vi "数字量输出配置.vi"() -> ()   [LabVIEW 2010] (continued)
            }
            frame 65 {
              w158 = TRUE
              w159 = FALSE ("单选_第41路")
              n5551 = local write "单选_第1路"(w158) -> ()
              n5552 = local write "单选_第2路"(w158) -> ()
              n5553 = local write "单选_第3路"(w158) -> ()
              n5554 = local write "单选_第4路"(w158) -> ()
              n5555 = local write "单选_第5路"(w158) -> ()
              n5556 = local write "单选_第6路"(w158) -> ()
              n5557 = local write "单选_第7路"(w158) -> ()
              n5558 = local write "单选_第8路"(w158) -> ()
              n5559 = local write "单选_第9路"(w158) -> ()
              n5560 = local write "单选_第10路"(w158) -> ()
              n5561 = local write "单选_第11路"(w158) -> ()
              n5562 = local write "单选_第12路"(w158) -> ()
              n5563 = local write "单选_第13路"(w158) -> ()
              n5564 = local write "单选_第14路"(w158) -> ()
              n5565 = local write "单选_第15路"(w158) -> ()
              n5566 = local write "单选_第16路"(w158) -> ()
              n5567 = local write "单选_第17路"(w158) -> ()
              n5568 = local write "单选_第18路"(w158) -> ()
              n5569 = local write "单选_第19路"(w158) -> ()
              n5570 = local write "单选_第20路"(w158) -> ()
              n5571 = local write "单选_第21路"(w158) -> ()
              n5572 = local write "单选_第22路"(w158) -> ()
              n5573 = local write "单选_第23路"(w158) -> ()
              n5574 = local write "单选_第24路"(w158) -> ()
              n5575 = local write "单选_第25路"(w158) -> ()
              n5576 = local write "单选_第26路"(w158) -> ()
              n5577 = local write "单选_第27路"(w158) -> ()
              n5578 = local write "单选_第28路"(w158) -> ()
              n5579 = local write "单选_第29路"(w158) -> ()
              n5580 = local write "单选_第30路"(w158) -> ()
              n5581 = local write "单选_第31路"(w158) -> ()
              n5582 = local write "单选_第32路"(w158) -> ()
              n5583 = local write "单选_第33路"(w158) -> ()
              n5584 = local write "单选_第34路"(w158) -> ()
              n5585 = local write "单选_第35路"(w158) -> ()
              n5586 = local write "单选_第36路"(w158) -> ()
              n5587 = local write "单选_第37路"(w158) -> ()
              n5588 = local write "单选_第38路"(w158) -> ()
              n5589 = local write "单选_第39路"(w158) -> ()
              n5590 = local write "单选_第40路"(w158) -> ()
              n5591 = local write "单选_第41路"(w158) -> ()
              n5592 = local write "单选_第42路"(w158) -> ()
              n5593 = local write "单选_第43路"(w158) -> ()
              n5594 = local write "单选_第44路"(w158) -> ()
              n5595 = local write "单选_第45路"(w158) -> ()
              n5596 = local write "单选_第46路"(w158) -> ()
              n5597 = local write "单选_第47路"(w158) -> ()
              n5598 = local write "单选_第48路"(w158) -> ()
              n5599 = local write "单选_第49路"(w158) -> ()
              n5600 = local write "单选_第50路"(w158) -> ()
              n5601 = local write "单选_第51路"(w158) -> ()
              n5602 = local write "单选_第52路"(w158) -> ()
              n5603 = local write "单选_第53路"(w158) -> ()
              n5604 = local write "单选_第54路"(w158) -> ()
              n5605 = local write "单选_第55路"(w158) -> ()
              n5606 = local write "单选_第56路"(w158) -> ()
              n5607 = local write "单选_第57路"(w158) -> ()
              n5608 = local write "单选_第58路"(w158) -> ()
              n5609 = local write "单选_第59路"(w158) -> ()
              n5610 = local write "单选_第60路"(w158) -> ()
              n5611 = local write "单选_第71路"(w159) -> ()
              n5612 = local write "单选_第79路"(w159) -> ()
              n5613 = local write "单选_第65路"(w158) -> ()
              n5614 = local write "单选_第66路"(w158) -> ()
              n5615 = local write "单选_第67路"(w158) -> ()
              n5616 = local write "单选_第68路"(w158) -> ()
              n5617 = local write "单选_第69路"(w158) -> ()
              n5618 = local write "单选_第70路"(w159) -> ()
              n5619 = local write "单选_第72路"(w159) -> ()
              n5620 = local write "单选_第73路"(w159) -> ()
              n5621 = local write "单选_第74路"(w159) -> ()
              n5622 = local write "单选_第75路"(w159) -> ()
              n5623 = local write "单选_第76路"(w159) -> ()
              n5624 = local write "单选_第77路"(w159) -> ()
              n5625 = local write "单选_第78路"(w159) -> ()
              n5626 = local write "单选_第80路"(w159) -> ()
            }
            frame 66 {
              w160 = TRUE
              w161 = FALSE ("单选_第41路")
              n5627 = local write "单选_第1路"(w160) -> ()
              n5628 = local write "单选_第2路"(w160) -> ()
              n5629 = local write "单选_第3路"(w160) -> ()
              n5630 = local write "单选_第4路"(w160) -> ()
              n5631 = local write "单选_第5路"(w160) -> ()
              n5632 = local write "单选_第6路"(w160) -> ()
              n5633 = local write "单选_第7路"(w160) -> ()
              n5634 = local write "单选_第8路"(w160) -> ()
              n5635 = local write "单选_第9路"(w160) -> ()
              n5636 = local write "单选_第10路"(w160) -> ()
              n5637 = local write "单选_第11路"(w160) -> ()
              n5638 = local write "单选_第12路"(w160) -> ()
              n5639 = local write "单选_第13路"(w160) -> ()
              n5640 = local write "单选_第14路"(w160) -> ()
              n5641 = local write "单选_第15路"(w160) -> ()
              n5642 = local write "单选_第16路"(w160) -> ()
              n5643 = local write "单选_第17路"(w160) -> ()
              n5644 = local write "单选_第18路"(w160) -> ()
              n5645 = local write "单选_第19路"(w160) -> ()
              n5646 = local write "单选_第20路"(w160) -> ()
              n5647 = local write "单选_第21路"(w160) -> ()
              n5648 = local write "单选_第22路"(w160) -> ()
              n5649 = local write "单选_第23路"(w160) -> ()
              n5650 = local write "单选_第24路"(w160) -> ()
              n5651 = local write "单选_第25路"(w160) -> ()
              n5652 = local write "单选_第26路"(w160) -> ()
              n5653 = local write "单选_第27路"(w160) -> ()
              n5654 = local write "单选_第28路"(w160) -> ()
              n5655 = local write "单选_第29路"(w160) -> ()
              n5656 = local write "单选_第30路"(w160) -> ()
              n5657 = local write "单选_第31路"(w160) -> ()
              n5658 = local write "单选_第32路"(w160) -> ()
              n5659 = local write "单选_第33路"(w160) -> ()
              n5660 = local write "单选_第34路"(w160) -> ()
              n5661 = local write "单选_第35路"(w160) -> ()
              n5662 = local write "单选_第36路"(w160) -> ()
              n5663 = local write "单选_第37路"(w160) -> ()
              n5664 = local write "单选_第38路"(w160) -> ()
              n5665 = local write "单选_第39路"(w160) -> ()
              n5666 = local write "单选_第40路"(w160) -> ()
              n5667 = local write "单选_第41路"(w160) -> ()
              n5668 = local write "单选_第42路"(w160) -> ()
              n5669 = local write "单选_第43路"(w160) -> ()
              n5670 = local write "单选_第44路"(w160) -> ()
              n5671 = local write "单选_第45路"(w160) -> ()
              n5672 = local write "单选_第46路"(w160) -> ()
              n5673 = local write "单选_第47路"(w160) -> ()
              n5674 = local write "单选_第48路"(w160) -> ()
              n5675 = local write "单选_第49路"(w160) -> ()
              n5676 = local write "单选_第50路"(w160) -> ()
              n5677 = local write "单选_第51路"(w160) -> ()
              n5678 = local write "单选_第52路"(w160) -> ()
              n5679 = local write "单选_第53路"(w160) -> ()
              n5680 = local write "单选_第54路"(w160) -> ()
              n5681 = local write "单选_第55路"(w160) -> ()
              n5682 = local write "单选_第56路"(w160) -> ()
              n5683 = local write "单选_第57路"(w160) -> ()
              n5684 = local write "单选_第58路"(w160) -> ()
              n5685 = local write "单选_第59路"(w160) -> ()
              n5686 = local write "单选_第60路"(w160) -> ()
              n5687 = local write "单选_第71路"(w161) -> ()
              n5688 = local write "单选_第79路"(w161) -> ()
              n5689 = local write "单选_第65路"(w160) -> ()
              n5690 = local write "单选_第66路"(w160) -> ()
              n5691 = local write "单选_第67路"(w160) -> ()
              n5692 = local write "单选_第68路"(w160) -> ()
              n5693 = local write "单选_第69路"(w160) -> ()
              n5694 = local write "单选_第70路"(w160) -> ()
              n5695 = local write "单选_第72路"(w161) -> ()
              n5696 = local write "单选_第73路"(w161) -> ()
              n5697 = local write "单选_第74路"(w161) -> ()
              n5698 = local write "单选_第75路"(w161) -> ()
              n5699 = local write "单选_第76路"(w161) -> ()
              n5700 = local write "单选_第77路"(w161) -> ()
              n5701 = local write "单选_第78路"(w161) -> ()
              n5702 = local write "单选_第80路"(w161) -> ()
            }
            frame 67 {
              w162 = TRUE
              w163 = FALSE ("单选_第41路")
              n5703 = local write "单选_第1路"(w162) -> ()
              n5704 = local write "单选_第2路"(w162) -> ()
              n5705 = local write "单选_第3路"(w162) -> ()
              n5706 = local write "单选_第4路"(w162) -> ()
              n5707 = local write "单选_第5路"(w162) -> ()
              n5708 = local write "单选_第6路"(w162) -> ()
              n5709 = local write "单选_第7路"(w162) -> ()
              n5710 = local write "单选_第8路"(w162) -> ()
              n5711 = local write "单选_第9路"(w162) -> ()
              n5712 = local write "单选_第10路"(w162) -> ()
              n5713 = local write "单选_第11路"(w162) -> ()
              n5714 = local write "单选_第12路"(w162) -> ()
              n5715 = local write "单选_第13路"(w162) -> ()
              n5716 = local write "单选_第14路"(w162) -> ()
              n5717 = local write "单选_第15路"(w162) -> ()
              n5718 = local write "单选_第16路"(w162) -> ()
              n5719 = local write "单选_第17路"(w162) -> ()
              n5720 = local write "单选_第18路"(w162) -> ()
              n5721 = local write "单选_第19路"(w162) -> ()
              n5722 = local write "单选_第20路"(w162) -> ()
              n5723 = local write "单选_第21路"(w162) -> ()
              n5724 = local write "单选_第22路"(w162) -> ()
              n5725 = local write "单选_第23路"(w162) -> ()
              n5726 = local write "单选_第24路"(w162) -> ()
              n5727 = local write "单选_第25路"(w162) -> ()
              n5728 = local write "单选_第26路"(w162) -> ()
              n5729 = local write "单选_第27路"(w162) -> ()
              n5730 = local write "单选_第28路"(w162) -> ()
              n5731 = local write "单选_第29路"(w162) -> ()
              n5732 = local write "单选_第30路"(w162) -> ()
              n5733 = local write "单选_第31路"(w162) -> ()
              n5734 = local write "单选_第32路"(w162) -> ()
              n5735 = local write "单选_第33路"(w162) -> ()
              n5736 = local write "单选_第34路"(w162) -> ()
              n5737 = local write "单选_第35路"(w162) -> ()
              n5738 = local write "单选_第36路"(w162) -> ()
              n5739 = local write "单选_第37路"(w162) -> ()
              n5740 = local write "单选_第38路"(w162) -> ()
              n5741 = local write "单选_第39路"(w162) -> ()
              n5742 = local write "单选_第40路"(w162) -> ()
              n5743 = local write "单选_第41路"(w162) -> ()
              n5744 = local write "单选_第42路"(w162) -> ()
              n5745 = local write "单选_第43路"(w162) -> ()
              n5746 = local write "单选_第44路"(w162) -> ()
              n5747 = local write "单选_第45路"(w162) -> ()
              n5748 = local write "单选_第46路"(w162) -> ()
              n5749 = local write "单选_第47路"(w162) -> ()
              n5750 = local write "单选_第48路"(w162) -> ()
              n5751 = local write "单选_第49路"(w162) -> ()
              n5752 = local write "单选_第50路"(w162) -> ()
              n5753 = local write "单选_第51路"(w162) -> ()
              n5754 = local write "单选_第52路"(w162) -> ()
              n5755 = local write "单选_第53路"(w162) -> ()
              n5756 = local write "单选_第54路"(w162) -> ()
              n5757 = local write "单选_第55路"(w162) -> ()
              n5758 = local write "单选_第56路"(w162) -> ()
              n5759 = local write "单选_第57路"(w162) -> ()
              n5760 = local write "单选_第58路"(w162) -> ()
              n5761 = local write "单选_第59路"(w162) -> ()
              n5762 = local write "单选_第60路"(w162) -> ()
              n5763 = local write "单选_第71路"(w162) -> ()
              n5764 = local write "单选_第79路"(w163) -> ()
              n5765 = local write "单选_第65路"(w162) -> ()
              n5766 = local write "单选_第66路"(w162) -> ()
              n5767 = local write "单选_第67路"(w162) -> ()
              n5768 = local write "单选_第68路"(w162) -> ()
              n5769 = local write "单选_第69路"(w162) -> ()
              n5770 = local write "单选_第70路"(w162) -> ()
              n5771 = local write "单选_第72路"(w163) -> ()
              n5772 = local write "单选_第73路"(w163) -> ()
              n5773 = local write "单选_第74路"(w163) -> ()
              n5774 = local write "单选_第75路"(w163) -> ()
              n5775 = local write "单选_第76路"(w163) -> ()
              n5776 = local write "单选_第77路"(w163) -> ()
              n5777 = local write "单选_第78路"(w163) -> ()
              n5778 = local write "单选_第80路"(w163) -> ()
            }
            frame 68 {
              w164 = TRUE
              w165 = FALSE ("单选_第41路")
              n5779 = local write "单选_第1路"(w164) -> ()
              n5780 = local write "单选_第2路"(w164) -> ()
              n5781 = local write "单选_第3路"(w164) -> ()
              n5782 = local write "单选_第4路"(w164) -> ()
              n5783 = local write "单选_第5路"(w164) -> ()
              n5784 = local write "单选_第6路"(w164) -> ()
              n5785 = local write "单选_第7路"(w164) -> ()
              n5786 = local write "单选_第8路"(w164) -> ()
              n5787 = local write "单选_第9路"(w164) -> ()
              n5788 = local write "单选_第10路"(w164) -> ()
              n5789 = local write "单选_第11路"(w164) -> ()
              n5790 = local write "单选_第12路"(w164) -> ()
              n5791 = local write "单选_第13路"(w164) -> ()
              n5792 = local write "单选_第14路"(w164) -> ()
              n5793 = local write "单选_第15路"(w164) -> ()
              n5794 = local write "单选_第16路"(w164) -> ()
              n5795 = local write "单选_第17路"(w164) -> ()
              n5796 = local write "单选_第18路"(w164) -> ()
              n5797 = local write "单选_第19路"(w164) -> ()
              n5798 = local write "单选_第20路"(w164) -> ()
              n5799 = local write "单选_第21路"(w164) -> ()
              n5800 = local write "单选_第22路"(w164) -> ()
              n5801 = local write "单选_第23路"(w164) -> ()
              n5802 = local write "单选_第24路"(w164) -> ()
              n5803 = local write "单选_第25路"(w164) -> ()
              n5804 = local write "单选_第26路"(w164) -> ()
              n5805 = local write "单选_第27路"(w164) -> ()
              n5806 = local write "单选_第28路"(w164) -> ()
              n5807 = local write "单选_第29路"(w164) -> ()
              n5808 = local write "单选_第30路"(w164) -> ()
              n5809 = local write "单选_第31路"(w164) -> ()
              n5810 = local write "单选_第32路"(w164) -> ()
              n5811 = local write "单选_第33路"(w164) -> ()
              n5812 = local write "单选_第34路"(w164) -> ()
              n5813 = local write "单选_第35路"(w164) -> ()
              n5814 = local write "单选_第36路"(w164) -> ()
              n5815 = local write "单选_第37路"(w164) -> ()
              n5816 = local write "单选_第38路"(w164) -> ()
              n5817 = local write "单选_第39路"(w164) -> ()
              n5818 = local write "单选_第40路"(w164) -> ()
              n5819 = local write "单选_第41路"(w164) -> ()
              n5820 = local write "单选_第42路"(w164) -> ()
              n5821 = local write "单选_第43路"(w164) -> ()
              n5822 = local write "单选_第44路"(w164) -> ()
              n5823 = local write "单选_第45路"(w164) -> ()
              n5824 = local write "单选_第46路"(w164) -> ()
              n5825 = local write "单选_第47路"(w164) -> ()
              n5826 = local write "单选_第48路"(w164) -> ()
              n5827 = local write "单选_第49路"(w164) -> ()
              n5828 = local write "单选_第50路"(w164) -> ()
              n5829 = local write "单选_第51路"(w164) -> ()
              n5830 = local write "单选_第52路"(w164) -> ()
              n5831 = local write "单选_第53路"(w164) -> ()
              n5832 = local write "单选_第54路"(w164) -> ()
              n5833 = local write "单选_第55路"(w164) -> ()
              n5834 = local write "单选_第56路"(w164) -> ()
              n5835 = local write "单选_第57路"(w164) -> ()
              n5836 = local write "单选_第58路"(w164) -> ()
              n5837 = local write "单选_第59路"(w164) -> ()
              n5838 = local write "单选_第60路"(w164) -> ()
              n5839 = local write "单选_第71路"(w164) -> ()
              n5840 = local write "单选_第79路"(w165) -> ()
              n5841 = local write "单选_第65路"(w164) -> ()
              n5842 = local write "单选_第66路"(w164) -> ()
              n5843 = local write "单选_第67路"(w164) -> ()
              n5844 = local write "单选_第68路"(w164) -> ()
              n5845 = local write "单选_第69路"(w164) -> ()
              n5846 = local write "单选_第70路"(w164) -> ()
              n5847 = local write "单选_第72路"(w164) -> ()
              n5848 = local write "单选_第73路"(w165) -> ()
              n5849 = local write "单选_第74路"(w165) -> ()
              n5850 = local write "单选_第75路"(w165) -> ()
              n5851 = local write "单选_第76路"(w165) -> ()
              n5852 = local write "单选_第77路"(w165) -> ()
              n5853 = local write "单选_第78路"(w165) -> ()
              n5854 = local write "单选_第80路"(w165) -> ()
            }
            frame 69 {
              w166 = TRUE
              w167 = FALSE ("单选_第41路")
              n5855 = local write "单选_第1路"(w166) -> ()
              n5856 = local write "单选_第2路"(w166) -> ()
              n5857 = local write "单选_第3路"(w166) -> ()
              n5858 = local write "单选_第4路"(w166) -> ()
              n5859 = local write "单选_第5路"(w166) -> ()
              n5860 = local write "单选_第6路"(w166) -> ()
              n5861 = local write "单选_第7路"(w166) -> ()
              n5862 = local write "单选_第8路"(w166) -> ()
              n5863 = local write "单选_第9路"(w166) -> ()
              n5864 = local write "单选_第10路"(w166) -> ()
              n5865 = local write "单选_第11路"(w166) -> ()
              n5866 = local write "单选_第12路"(w166) -> ()
              n5867 = local write "单选_第13路"(w166) -> ()
              n5868 = local write "单选_第14路"(w166) -> ()
              n5869 = local write "单选_第15路"(w166) -> ()
              n5870 = local write "单选_第16路"(w166) -> ()
              n5871 = local write "单选_第17路"(w166) -> ()
              n5872 = local write "单选_第18路"(w166) -> ()
              n5873 = local write "单选_第19路"(w166) -> ()
              n5874 = local write "单选_第20路"(w166) -> ()
              n5875 = local write "单选_第21路"(w166) -> ()
              n5876 = local write "单选_第22路"(w166) -> ()
              n5877 = local write "单选_第23路"(w166) -> ()
              n5878 = local write "单选_第24路"(w166) -> ()
              n5879 = local write "单选_第25路"(w166) -> ()
              n5880 = local write "单选_第26路"(w166) -> ()
              n5881 = local write "单选_第27路"(w166) -> ()
              n5882 = local write "单选_第28路"(w166) -> ()
              n5883 = local write "单选_第29路"(w166) -> ()
              n5884 = local write "单选_第30路"(w166) -> ()
              n5885 = local write "单选_第31路"(w166) -> ()
              n5886 = local write "单选_第32路"(w166) -> ()
              n5887 = local write "单选_第33路"(w166) -> ()
              n5888 = local write "单选_第34路"(w166) -> ()
              n5889 = local write "单选_第35路"(w166) -> ()
              n5890 = local write "单选_第36路"(w166) -> ()
              n5891 = local write "单选_第37路"(w166) -> ()
              n5892 = local write "单选_第38路"(w166) -> ()
              n5893 = local write "单选_第39路"(w166) -> ()
              n5894 = local write "单选_第40路"(w166) -> ()
              n5895 = local write "单选_第41路"(w166) -> ()
              n5896 = local write "单选_第42路"(w166) -> ()
              n5897 = local write "单选_第43路"(w166) -> ()
              n5898 = local write "单选_第44路"(w166) -> ()
              n5899 = local write "单选_第45路"(w166) -> ()
              n5900 = local write "单选_第46路"(w166) -> ()
              n5901 = local write "单选_第47路"(w166) -> ()
              n5902 = local write "单选_第48路"(w166) -> ()
              n5903 = local write "单选_第49路"(w166) -> ()
              n5904 = local write "单选_第50路"(w166) -> ()
              n5905 = local write "单选_第51路"(w166) -> ()
              n5906 = local write "单选_第52路"(w166) -> ()
              n5907 = local write "单选_第53路"(w166) -> ()
              n5908 = local write "单选_第54路"(w166) -> ()
              n5909 = local write "单选_第55路"(w166) -> ()
              n5910 = local write "单选_第56路"(w166) -> ()
              n5911 = local write "单选_第57路"(w166) -> ()
              n5912 = local write "单选_第58路"(w166) -> ()
              n5913 = local write "单选_第59路"(w166) -> ()
              n5914 = local write "单选_第60路"(w166) -> ()
              n5915 = local write "单选_第71路"(w166) -> ()
              n5916 = local write "单选_第79路"(w167) -> ()
              n5917 = local write "单选_第65路"(w166) -> ()
              n5918 = local write "单选_第66路"(w166) -> ()
              n5919 = local write "单选_第67路"(w166) -> ()
              n5920 = local write "单选_第68路"(w166) -> ()
              n5921 = local write "单选_第69路"(w166) -> ()
              n5922 = local write "单选_第70路"(w166) -> ()
              n5923 = local write "单选_第72路"(w166) -> ()
              n5924 = local write "单选_第73路"(w166) -> ()
              n5925 = local write "单选_第74路"(w167) -> ()
              n5926 = local write "单选_第75路"(w167) -> ()
              n5927 = local write "单选_第76路"(w167) -> ()
              n5928 = local write "单选_第77路"(w167) -> ()
              n5929 = local write "单选_第78路"(w167) -> ()
              n5930 = local write "单选_第80路"(w167) -> ()
            }
            frame 70 {
              w168 = TRUE
              w169 = FALSE ("单选_第41路")
              n5931 = local write "单选_第1路"(w168) -> ()
              n5932 = local write "单选_第2路"(w168) -> ()
              n5933 = local write "单选_第3路"(w168) -> ()
              n5934 = local write "单选_第4路"(w168) -> ()
              n5935 = local write "单选_第5路"(w168) -> ()
              n5936 = local write "单选_第6路"(w168) -> ()
              n5937 = local write "单选_第7路"(w168) -> ()
              n5938 = local write "单选_第8路"(w168) -> ()
              n5939 = local write "单选_第9路"(w168) -> ()
              n5940 = local write "单选_第10路"(w168) -> ()
              n5941 = local write "单选_第11路"(w168) -> ()
              n5942 = local write "单选_第12路"(w168) -> ()
              n5943 = local write "单选_第13路"(w168) -> ()
              n5944 = local write "单选_第14路"(w168) -> ()
              n5945 = local write "单选_第15路"(w168) -> ()
              n5946 = local write "单选_第16路"(w168) -> ()
              n5947 = local write "单选_第17路"(w168) -> ()
              n5948 = local write "单选_第18路"(w168) -> ()
              n5949 = local write "单选_第19路"(w168) -> ()
              n5950 = local write "单选_第20路"(w168) -> ()
              n5951 = local write "单选_第21路"(w168) -> ()
              n5952 = local write "单选_第22路"(w168) -> ()
              n5953 = local write "单选_第23路"(w168) -> ()
              n5954 = local write "单选_第24路"(w168) -> ()
              n5955 = local write "单选_第25路"(w168) -> ()
              n5956 = local write "单选_第26路"(w168) -> ()
              n5957 = local write "单选_第27路"(w168) -> ()
              n5958 = local write "单选_第28路"(w168) -> ()
              n5959 = local write "单选_第29路"(w168) -> ()
              n5960 = local write "单选_第30路"(w168) -> ()
              n5961 = local write "单选_第31路"(w168) -> ()
              n5962 = local write "单选_第32路"(w168) -> ()
              n5963 = local write "单选_第33路"(w168) -> ()
              n5964 = local write "单选_第34路"(w168) -> ()
              n5965 = local write "单选_第35路"(w168) -> ()
              n5966 = local write "单选_第36路"(w168) -> ()
              n5967 = local write "单选_第37路"(w168) -> ()
              n5968 = local write "单选_第38路"(w168) -> ()
              n5969 = local write "单选_第39路"(w168) -> ()
              n5970 = local write "单选_第40路"(w168) -> ()
              n5971 = local write "单选_第41路"(w168) -> ()
              n5972 = local write "单选_第42路"(w168) -> ()
              n5973 = local write "单选_第43路"(w168) -> ()
              n5974 = local write "单选_第44路"(w168) -> ()
              n5975 = local write "单选_第45路"(w168) -> ()
              n5976 = local write "单选_第46路"(w168) -> ()
              n5977 = local write "单选_第47路"(w168) -> ()
              n5978 = local write "单选_第48路"(w168) -> ()
              n5979 = local write "单选_第49路"(w168) -> ()
              n5980 = local write "单选_第50路"(w168) -> ()
              n5981 = local write "单选_第51路"(w168) -> ()
              n5982 = local write "单选_第52路"(w168) -> ()
              n5983 = local write "单选_第53路"(w168) -> ()
              n5984 = local write "单选_第54路"(w168) -> ()
              n5985 = local write "单选_第55路"(w168) -> ()
              n5986 = local write "单选_第56路"(w168) -> ()
              n5987 = local write "单选_第57路"(w168) -> ()
              n5988 = local write "单选_第58路"(w168) -> ()
              n5989 = local write "单选_第59路"(w168) -> ()
              n5990 = local write "单选_第60路"(w168) -> ()
              n5991 = local write "单选_第71路"(w168) -> ()
              n5992 = local write "单选_第79路"(w169) -> ()
              n5993 = local write "单选_第65路"(w168) -> ()
              n5994 = local write "单选_第66路"(w168) -> ()
              n5995 = local write "单选_第67路"(w168) -> ()
              n5996 = local write "单选_第68路"(w168) -> ()
              n5997 = local write "单选_第69路"(w168) -> ()
              n5998 = local write "单选_第70路"(w168) -> ()
              n5999 = local write "单选_第72路"(w168) -> ()
              n6000 = local write "单选_第73路"(w168) -> ()
              n6001 = local write "单选_第74路"(w168) -> ()
              n6002 = local write "单选_第75路"(w169) -> ()
              n6003 = local write "单选_第76路"(w169) -> ()
              n6004 = local write "单选_第77路"(w169) -> ()
              n6005 = local write "单选_第78路"(w169) -> ()
              n6006 = local write "单选_第80路"(w169) -> ()
            }
            frame 71 {
              w170 = TRUE
              w171 = FALSE ("单选_第41路")
              n6007 = local write "单选_第1路"(w170) -> ()
              n6008 = local write "单选_第2路"(w170) -> ()
              n6009 = local write "单选_第3路"(w170) -> ()
              n6010 = local write "单选_第4路"(w170) -> ()
              n6011 = local write "单选_第5路"(w170) -> ()
              n6012 = local write "单选_第6路"(w170) -> ()
              n6013 = local write "单选_第7路"(w170) -> ()
              n6014 = local write "单选_第8路"(w170) -> ()
              n6015 = local write "单选_第9路"(w170) -> ()
              n6016 = local write "单选_第10路"(w170) -> ()
              n6017 = local write "单选_第11路"(w170) -> ()
              n6018 = local write "单选_第12路"(w170) -> ()
              n6019 = local write "单选_第13路"(w170) -> ()
              n6020 = local write "单选_第14路"(w170) -> ()
              n6021 = local write "单选_第15路"(w170) -> ()
              n6022 = local write "单选_第16路"(w170) -> ()
              n6023 = local write "单选_第17路"(w170) -> ()
              n6024 = local write "单选_第18路"(w170) -> ()
              n6025 = local write "单选_第19路"(w170) -> ()
              n6026 = local write "单选_第20路"(w170) -> ()
              n6027 = local write "单选_第21路"(w170) -> ()
              n6028 = local write "单选_第22路"(w170) -> ()
              n6029 = local write "单选_第23路"(w170) -> ()
              n6030 = local write "单选_第24路"(w170) -> ()
              n6031 = local write "单选_第25路"(w170) -> ()
              n6032 = local write "单选_第26路"(w170) -> ()
              n6033 = local write "单选_第27路"(w170) -> ()
              n6034 = local write "单选_第28路"(w170) -> ()
              n6035 = local write "单选_第29路"(w170) -> ()
              n6036 = local write "单选_第30路"(w170) -> ()
              n6037 = local write "单选_第31路"(w170) -> ()
              n6038 = local write "单选_第32路"(w170) -> ()
              n6039 = local write "单选_第33路"(w170) -> ()
              n6040 = local write "单选_第34路"(w170) -> ()
              n6041 = local write "单选_第35路"(w170) -> ()
              n6042 = local write "单选_第36路"(w170) -> ()
              n6043 = local write "单选_第37路"(w170) -> ()
              n6044 = local write "单选_第38路"(w170) -> ()
              n6045 = local write "单选_第39路"(w170) -> ()
              n6046 = local write "单选_第40路"(w170) -> ()
              n6047 = local write "单选_第41路"(w170) -> ()
              n6048 = local write "单选_第42路"(w170) -> ()
              n6049 = local write "单选_第43路"(w170) -> ()
              n6050 = local write "单选_第44路"(w170) -> ()
              n6051 = local write "单选_第45路"(w170) -> ()
              n6052 = local write "单选_第46路"(w170) -> ()
              n6053 = local write "单选_第47路"(w170) -> ()
              n6054 = local write "单选_第48路"(w170) -> ()
              n6055 = local write "单选_第49路"(w170) -> ()
              n6056 = local write "单选_第50路"(w170) -> ()
              n6057 = local write "单选_第51路"(w170) -> ()
              n6058 = local write "单选_第52路"(w170) -> ()
              n6059 = local write "单选_第53路"(w170) -> ()
              n6060 = local write "单选_第54路"(w170) -> ()
              n6061 = local write "单选_第55路"(w170) -> ()
              n6062 = local write "单选_第56路"(w170) -> ()
              n6063 = local write "单选_第57路"(w170) -> ()
              n6064 = local write "单选_第58路"(w170) -> ()
              n6065 = local write "单选_第59路"(w170) -> ()
              n6066 = local write "单选_第60路"(w170) -> ()
              n6067 = local write "单选_第71路"(w170) -> ()
              n6068 = local write "单选_第79路"(w171) -> ()
              n6069 = local write "单选_第65路"(w170) -> ()
              n6070 = local write "单选_第66路"(w170) -> ()
              n6071 = local write "单选_第67路"(w170) -> ()
              n6072 = local write "单选_第68路"(w170) -> ()
              n6073 = local write "单选_第69路"(w170) -> ()
              n6074 = local write "单选_第70路"(w170) -> ()
              n6075 = local write "单选_第72路"(w170) -> ()
              n6076 = local write "单选_第73路"(w170) -> ()
              n6077 = local write "单选_第74路"(w170) -> ()
              n6078 = local write "单选_第75路"(w170) -> ()
              n6079 = local write "单选_第76路"(w171) -> ()
              n6080 = local write "单选_第77路"(w171) -> ()
              n6081 = local write "单选_第78路"(w171) -> ()
              n6082 = local write "单选_第80路"(w171) -> ()
            }
            frame 72 {
              w172 = TRUE
              w173 = FALSE ("单选_第41路")
              n6083 = local write "单选_第1路"(w172) -> ()
              n6084 = local write "单选_第2路"(w172) -> ()
              n6085 = local write "单选_第3路"(w172) -> ()
              n6086 = local write "单选_第4路"(w172) -> ()
              n6087 = local write "单选_第5路"(w172) -> ()
              n6088 = local write "单选_第6路"(w172) -> ()
              n6089 = local write "单选_第7路"(w172) -> ()
              n6090 = local write "单选_第8路"(w172) -> ()
              n6091 = local write "单选_第9路"(w172) -> ()
              n6092 = local write "单选_第10路"(w172) -> ()
              n6093 = local write "单选_第11路"(w172) -> ()
              n6094 = local write "单选_第12路"(w172) -> ()
              n6095 = local write "单选_第13路"(w172) -> ()
              n6096 = local write "单选_第14路"(w172) -> ()
              n6097 = local write "单选_第15路"(w172) -> ()
              n6098 = local write "单选_第16路"(w172) -> ()
              n6099 = local write "单选_第17路"(w172) -> ()
              n6100 = local write "单选_第18路"(w172) -> ()
              n6101 = local write "单选_第19路"(w172) -> ()
              n6102 = local write "单选_第20路"(w172) -> ()
              n6103 = local write "单选_第21路"(w172) -> ()
              n6104 = local write "单选_第22路"(w172) -> ()
              n6105 = local write "单选_第23路"(w172) -> ()
              n6106 = local write "单选_第24路"(w172) -> ()
              n6107 = local write "单选_第25路"(w172) -> ()
              n6108 = local write "单选_第26路"(w172) -> ()
              n6109 = local write "单选_第27路"(w172) -> ()
              n6110 = local write "单选_第28路"(w172) -> ()
              n6111 = local write "单选_第29路"(w172) -> ()
              n6112 = local write "单选_第30路"(w172) -> ()
              n6113 = local write "单选_第31路"(w172) -> ()
              n6114 = local write "单选_第32路"(w172) -> ()
              n6115 = local write "单选_第33路"(w172) -> ()
              n6116 = local write "单选_第34路"(w172) -> ()
              n6117 = local write "单选_第35路"(w172) -> ()
              n6118 = local write "单选_第36路"(w172) -> ()
              n6119 = local write "单选_第37路"(w172) -> ()
              n6120 = local write "单选_第38路"(w172) -> ()
              n6121 = local write "单选_第39路"(w172) -> ()
              n6122 = local write "单选_第40路"(w172) -> ()
              n6123 = local write "单选_第41路"(w172) -> ()
              n6124 = local write "单选_第42路"(w172) -> ()
              n6125 = local write "单选_第43路"(w172) -> ()
              n6126 = local write "单选_第44路"(w172) -> ()
              n6127 = local write "单选_第45路"(w172) -> ()
              n6128 = local write "单选_第46路"(w172) -> ()
              n6129 = local write "单选_第47路"(w172) -> ()
              n6130 = local write "单选_第48路"(w172) -> ()
              n6131 = local write "单选_第49路"(w172) -> ()
              n6132 = local write "单选_第50路"(w172) -> ()
              n6133 = local write "单选_第51路"(w172) -> ()
              n6134 = local write "单选_第52路"(w172) -> ()
              n6135 = local write "单选_第53路"(w172) -> ()
              n6136 = local write "单选_第54路"(w172) -> ()
              n6137 = local write "单选_第55路"(w172) -> ()
              n6138 = local write "单选_第56路"(w172) -> ()
              n6139 = local write "单选_第57路"(w172) -> ()
              n6140 = local write "单选_第58路"(w172) -> ()
              n6141 = local write "单选_第59路"(w172) -> ()
              n6142 = local write "单选_第60路"(w172) -> ()
              n6143 = local write "单选_第71路"(w172) -> ()
              n6144 = local write "单选_第79路"(w173) -> ()
              n6145 = local write "单选_第65路"(w172) -> ()
              n6146 = local write "单选_第66路"(w172) -> ()
              n6147 = local write "单选_第67路"(w172) -> ()
              n6148 = local write "单选_第68路"(w172) -> ()
              n6149 = local write "单选_第69路"(w172) -> ()
              n6150 = local write "单选_第70路"(w172) -> ()
              n6151 = local write "单选_第72路"(w172) -> ()
              n6152 = local write "单选_第73路"(w172) -> ()
              n6153 = local write "单选_第74路"(w172) -> ()
              n6154 = local write "单选_第75路"(w172) -> ()
              n6155 = local write "单选_第76路"(w172) -> ()
              n6156 = local write "单选_第77路"(w173) -> ()
              n6157 = local write "单选_第78路"(w173) -> ()
              n6158 = local write "单选_第80路"(w173) -> ()
            }
            frame 73 {
              w174 = TRUE
              w175 = FALSE ("单选_第41路")
              n6159 = local write "单选_第1路"(w174) -> ()
              n6160 = local write "单选_第2路"(w174) -> ()
              n6161 = local write "单选_第3路"(w174) -> ()
              n6162 = local write "单选_第4路"(w174) -> ()
              n6163 = local write "单选_第5路"(w174) -> ()
              n6164 = local write "单选_第6路"(w174) -> ()
              n6165 = local write "单选_第7路"(w174) -> ()
              n6166 = local write "单选_第8路"(w174) -> ()
              n6167 = local write "单选_第9路"(w174) -> ()
              n6168 = local write "单选_第10路"(w174) -> ()
              n6169 = local write "单选_第11路"(w174) -> ()
              n6170 = local write "单选_第12路"(w174) -> ()
              n6171 = local write "单选_第13路"(w174) -> ()
              n6172 = local write "单选_第14路"(w174) -> ()
              n6173 = local write "单选_第15路"(w174) -> ()
              n6174 = local write "单选_第16路"(w174) -> ()
              n6175 = local write "单选_第17路"(w174) -> ()
              n6176 = local write "单选_第18路"(w174) -> ()
              n6177 = local write "单选_第19路"(w174) -> ()
              n6178 = local write "单选_第20路"(w174) -> ()
              n6179 = local write "单选_第21路"(w174) -> ()
              n6180 = local write "单选_第22路"(w174) -> ()
              n6181 = local write "单选_第23路"(w174) -> ()
              n6182 = local write "单选_第24路"(w174) -> ()
              n6183 = local write "单选_第25路"(w174) -> ()
              n6184 = local write "单选_第26路"(w174) -> ()
              n6185 = local write "单选_第27路"(w174) -> ()
              n6186 = local write "单选_第28路"(w174) -> ()
              n6187 = local write "单选_第29路"(w174) -> ()
              n6188 = local write "单选_第30路"(w174) -> ()
              n6189 = local write "单选_第31路"(w174) -> ()
              n6190 = local write "单选_第32路"(w174) -> ()
              n6191 = local write "单选_第33路"(w174) -> ()
              n6192 = local write "单选_第34路"(w174) -> ()
              n6193 = local write "单选_第35路"(w174) -> ()
              n6194 = local write "单选_第36路"(w174) -> ()
              n6195 = local write "单选_第37路"(w174) -> ()
              n6196 = local write "单选_第38路"(w174) -> ()
              n6197 = local write "单选_第39路"(w174) -> ()
              n6198 = local write "单选_第40路"(w174) -> ()
              n6199 = local write "单选_第41路"(w174) -> ()
              n6200 = local write "单选_第42路"(w174) -> ()
              n6201 = local write "单选_第43路"(w174) -> ()
              n6202 = local write "单选_第44路"(w174) -> ()
              n6203 = local write "单选_第45路"(w174) -> ()
              n6204 = local write "单选_第46路"(w174) -> ()
              n6205 = local write "单选_第47路"(w174) -> ()
              n6206 = local write "单选_第48路"(w174) -> ()
              n6207 = local write "单选_第49路"(w174) -> ()
              n6208 = local write "单选_第50路"(w174) -> ()
              n6209 = local write "单选_第51路"(w174) -> ()
              n6210 = local write "单选_第52路"(w174) -> ()
              n6211 = local write "单选_第53路"(w174) -> ()
              n6212 = local write "单选_第54路"(w174) -> ()
              n6213 = local write "单选_第55路"(w174) -> ()
              n6214 = local write "单选_第56路"(w174) -> ()
              n6215 = local write "单选_第57路"(w174) -> ()
              n6216 = local write "单选_第58路"(w174) -> ()
              n6217 = local write "单选_第59路"(w174) -> ()
              n6218 = local write "单选_第60路"(w174) -> ()
              n6219 = local write "单选_第71路"(w174) -> ()
              n6220 = local write "单选_第79路"(w175) -> ()
              n6221 = local write "单选_第65路"(w174) -> ()
              n6222 = local write "单选_第66路"(w174) -> ()
              n6223 = local write "单选_第67路"(w174) -> ()
              n6224 = local write "单选_第68路"(w174) -> ()
              n6225 = local write "单选_第69路"(w174) -> ()
              n6226 = local write "单选_第70路"(w174) -> ()
              n6227 = local write "单选_第72路"(w174) -> ()
              n6228 = local write "单选_第73路"(w174) -> ()
              n6229 = local write "单选_第74路"(w174) -> ()
              n6230 = local write "单选_第75路"(w174) -> ()
              n6231 = local write "单选_第76路"(w174) -> ()
              n6232 = local write "单选_第77路"(w174) -> ()
              n6233 = local write "单选_第78路"(w175) -> ()
              n6234 = local write "单选_第80路"(w175) -> ()
            }
            frame 74 {
              w176 = TRUE
              w177 = FALSE ("单选_第41路")
              n6235 = local write "单选_第1路"(w176) -> ()
              n6236 = local write "单选_第2路"(w176) -> ()
              n6237 = local write "单选_第3路"(w176) -> ()
              n6238 = local write "单选_第4路"(w176) -> ()
              n6239 = local write "单选_第5路"(w176) -> ()
              n6240 = local write "单选_第6路"(w176) -> ()
              n6241 = local write "单选_第7路"(w176) -> ()
              n6242 = local write "单选_第8路"(w176) -> ()
              n6243 = local write "单选_第9路"(w176) -> ()
              n6244 = local write "单选_第10路"(w176) -> ()
              n6245 = local write "单选_第11路"(w176) -> ()
              n6246 = local write "单选_第12路"(w176) -> ()
              n6247 = local write "单选_第13路"(w176) -> ()
              n6248 = local write "单选_第14路"(w176) -> ()
              n6249 = local write "单选_第15路"(w176) -> ()
              n6250 = local write "单选_第16路"(w176) -> ()
              n6251 = local write "单选_第17路"(w176) -> ()
              n6252 = local write "单选_第18路"(w176) -> ()
              n6253 = local write "单选_第19路"(w176) -> ()
              n6254 = local write "单选_第20路"(w176) -> ()
              n6255 = local write "单选_第21路"(w176) -> ()
              n6256 = local write "单选_第22路"(w176) -> ()
              n6257 = local write "单选_第23路"(w176) -> ()
              n6258 = local write "单选_第24路"(w176) -> ()
              n6259 = local write "单选_第25路"(w176) -> ()
              n6260 = local write "单选_第26路"(w176) -> ()
              n6261 = local write "单选_第27路"(w176) -> ()
              n6262 = local write "单选_第28路"(w176) -> ()
              n6263 = local write "单选_第29路"(w176) -> ()
              n6264 = local write "单选_第30路"(w176) -> ()
              n6265 = local write "单选_第31路"(w176) -> ()
              n6266 = local write "单选_第32路"(w176) -> ()
              n6267 = local write "单选_第33路"(w176) -> ()
              n6268 = local write "单选_第34路"(w176) -> ()
              n6269 = local write "单选_第35路"(w176) -> ()
              n6270 = local write "单选_第36路"(w176) -> ()
              n6271 = local write "单选_第37路"(w176) -> ()
              n6272 = local write "单选_第38路"(w176) -> ()
              n6273 = local write "单选_第39路"(w176) -> ()
              n6274 = local write "单选_第40路"(w176) -> ()
              n6275 = local write "单选_第41路"(w176) -> ()
              n6276 = local write "单选_第42路"(w176) -> ()
              n6277 = local write "单选_第43路"(w176) -> ()
              n6278 = local write "单选_第44路"(w176) -> ()
              n6279 = local write "单选_第45路"(w176) -> ()
              n6280 = local write "单选_第46路"(w176) -> ()
              n6281 = local write "单选_第47路"(w176) -> ()
              n6282 = local write "单选_第48路"(w176) -> ()
              n6283 = local write "单选_第49路"(w176) -> ()
              n6284 = local write "单选_第50路"(w176) -> ()
              n6285 = local write "单选_第51路"(w176) -> ()
              n6286 = local write "单选_第52路"(w176) -> ()
              n6287 = local write "单选_第53路"(w176) -> ()
              n6288 = local write "单选_第54路"(w176) -> ()
              n6289 = local write "单选_第55路"(w176) -> ()
              n6290 = local write "单选_第56路"(w176) -> ()
              n6291 = local write "单选_第57路"(w176) -> ()
              n6292 = local write "单选_第58路"(w176) -> ()
              n6293 = local write "单选_第59路"(w176) -> ()
              n6294 = local write "单选_第60路"(w176) -> ()
              n6295 = local write "单选_第71路"(w176) -> ()
              n6296 = local write "单选_第79路"(w177) -> ()
              n6297 = local write "单选_第65路"(w176) -> ()
              n6298 = local write "单选_第66路"(w176) -> ()
              n6299 = local write "单选_第67路"(w176) -> ()
              n6300 = local write "单选_第68路"(w176) -> ()
              n6301 = local write "单选_第69路"(w176) -> ()
              n6302 = local write "单选_第70路"(w176) -> ()
              n6303 = local write "单选_第72路"(w176) -> ()
              n6304 = local write "单选_第73路"(w176) -> ()
              n6305 = local write "单选_第74路"(w176) -> ()
              n6306 = local write "单选_第75路"(w176) -> ()
              n6307 = local write "单选_第76路"(w176) -> ()
              n6308 = local write "单选_第77路"(w176) -> ()
              n6309 = local write "单选_第78路"(w176) -> ()
              n6310 = local write "单选_第80路"(w177) -> ()
            }
            frame 75 {
              w178 = TRUE
              n6311 = local write "单选_第1路"(w178) -> ()
              n6312 = local write "单选_第2路"(w178) -> ()
              n6313 = local write "单选_第3路"(w178) -> ()
              n6314 = local write "单选_第4路"(w178) -> ()
              n6315 = local write "单选_第5路"(w178) -> ()
              n6316 = local write "单选_第6路"(w178) -> ()
              n6317 = local write "单选_第7路"(w178) -> ()
              n6318 = local write "单选_第8路"(w178) -> ()
              n6319 = local write "单选_第9路"(w178) -> ()
              n6320 = local write "单选_第10路"(w178) -> ()
              n6321 = local write "单选_第11路"(w178) -> ()
              n6322 = local write "单选_第12路"(w178) -> ()
              n6323 = local write "单选_第13路"(w178) -> ()
              n6324 = local write "单选_第14路"(w178) -> ()
              n6325 = local write "单选_第15路"(w178) -> ()
              n6326 = local write "单选_第16路"(w178) -> ()
              n6327 = local write "单选_第17路"(w178) -> ()
              n6328 = local write "单选_第18路"(w178) -> ()
              n6329 = local write "单选_第19路"(w178) -> ()
              n6330 = local write "单选_第20路"(w178) -> ()
              n6331 = local write "单选_第21路"(w178) -> ()
              n6332 = local write "单选_第22路"(w178) -> ()
              n6333 = local write "单选_第23路"(w178) -> ()
              n6334 = local write "单选_第24路"(w178) -> ()
              n6335 = local write "单选_第25路"(w178) -> ()
              n6336 = local write "单选_第26路"(w178) -> ()
              n6337 = local write "单选_第27路"(w178) -> ()
              n6338 = local write "单选_第28路"(w178) -> ()
              n6339 = local write "单选_第29路"(w178) -> ()
              n6340 = local write "单选_第30路"(w178) -> ()
              n6341 = local write "单选_第31路"(w178) -> ()
              n6342 = local write "单选_第32路"(w178) -> ()
              n6343 = local write "单选_第33路"(w178) -> ()
              n6344 = local write "单选_第34路"(w178) -> ()
              n6345 = local write "单选_第35路"(w178) -> ()
              n6346 = local write "单选_第36路"(w178) -> ()
              n6347 = local write "单选_第37路"(w178) -> ()
              n6348 = local write "单选_第38路"(w178) -> ()
              n6349 = local write "单选_第39路"(w178) -> ()
              n6350 = local write "单选_第40路"(w178) -> ()
              n6351 = local write "单选_第41路"(w178) -> ()
              n6352 = local write "单选_第42路"(w178) -> ()
              n6353 = local write "单选_第43路"(w178) -> ()
              n6354 = local write "单选_第44路"(w178) -> ()
              n6355 = local write "单选_第45路"(w178) -> ()
              n6356 = local write "单选_第46路"(w178) -> ()
              n6357 = local write "单选_第47路"(w178) -> ()
              n6358 = local write "单选_第48路"(w178) -> ()
              n6359 = local write "单选_第49路"(w178) -> ()
              n6360 = local write "单选_第50路"(w178) -> ()
              n6361 = local write "单选_第51路"(w178) -> ()
              n6362 = local write "单选_第52路"(w178) -> ()
              n6363 = local write "单选_第53路"(w178) -> ()
              n6364 = local write "单选_第54路"(w178) -> ()
              n6365 = local write "单选_第55路"(w178) -> ()
              n6366 = local write "单选_第56路"(w178) -> ()
              n6367 = local write "单选_第57路"(w178) -> ()
              n6368 = local write "单选_第58路"(w178) -> ()
              n6369 = local write "单选_第59路"(w178) -> ()
              n6370 = local write "单选_第60路"(w178) -> ()
              n6371 = local write "单选_第71路"(w178) -> ()
              n6372 = local write "单选_第79路"(w178) -> ()
              n6373 = local write "单选_第65路"(w178) -> ()
              n6374 = local write "单选_第66路"(w178) -> ()
              n6375 = local write "单选_第67路"(w178) -> ()
              n6376 = local write "单选_第68路"(w178) -> ()
              n6377 = local write "单选_第69路"(w178) -> ()
              n6378 = local write "单选_第70路"(w178) -> ()
              n6379 = local write "单选_第72路"(w178) -> ()
              n6380 = local write "单选_第73路"(w178) -> ()
              n6381 = local write "单选_第74路"(w178) -> ()
              n6382 = local write "单选_第75路"(w178) -> ()
              n6383 = local write "单选_第76路"(w178) -> ()
              n6384 = local write "单选_第77路"(w178) -> ()
              n6385 = local write "单选_第78路"(w178) -> ()
              n6386 = local write "单选_第80路"(FALSE ("单选_第41路")) -> ()
            }
            frame 76 {
              w180 = TRUE
              n6387 = local write "单选_第1路"(w180) -> ()
              n6388 = local write "单选_第2路"(w180) -> ()
              n6389 = local write "单选_第3路"(w180) -> ()
              n6390 = local write "单选_第4路"(w180) -> ()
              n6391 = local write "单选_第5路"(w180) -> ()
              n6392 = local write "单选_第6路"(w180) -> ()
              n6393 = local write "单选_第7路"(w180) -> ()
              n6394 = local write "单选_第8路"(w180) -> ()
              n6395 = local write "单选_第9路"(w180) -> ()
              n6396 = local write "单选_第10路"(w180) -> ()
              n6397 = local write "单选_第11路"(w180) -> ()
              n6398 = local write "单选_第12路"(w180) -> ()
              n6399 = local write "单选_第13路"(w180) -> ()
              n6400 = local write "单选_第14路"(w180) -> ()
              n6401 = local write "单选_第15路"(w180) -> ()
              n6402 = local write "单选_第16路"(w180) -> ()
              n6403 = local write "单选_第17路"(w180) -> ()
              n6404 = local write "单选_第18路"(w180) -> ()
              n6405 = local write "单选_第19路"(w180) -> ()
              n6406 = local write "单选_第20路"(w180) -> ()
              n6407 = local write "单选_第21路"(w180) -> ()
              n6408 = local write "单选_第22路"(w180) -> ()
              n6409 = local write "单选_第23路"(w180) -> ()
              n6410 = local write "单选_第24路"(w180) -> ()
              n6411 = local write "单选_第25路"(w180) -> ()
              n6412 = local write "单选_第26路"(w180) -> ()
              n6413 = local write "单选_第27路"(w180) -> ()
              n6414 = local write "单选_第28路"(w180) -> ()
              n6415 = local write "单选_第29路"(w180) -> ()
              n6416 = local write "单选_第30路"(w180) -> ()
              n6417 = local write "单选_第31路"(w180) -> ()
              n6418 = local write "单选_第32路"(w180) -> ()
              n6419 = local write "单选_第33路"(w180) -> ()
              n6420 = local write "单选_第34路"(w180) -> ()
              n6421 = local write "单选_第35路"(w180) -> ()
              n6422 = local write "单选_第36路"(w180) -> ()
              n6423 = local write "单选_第37路"(w180) -> ()
              n6424 = local write "单选_第38路"(w180) -> ()
              n6425 = local write "单选_第39路"(w180) -> ()
              n6426 = local write "单选_第40路"(w180) -> ()
              n6427 = local write "单选_第41路"(w180) -> ()
              n6428 = local write "单选_第42路"(w180) -> ()
              n6429 = local write "单选_第43路"(w180) -> ()
              n6430 = local write "单选_第44路"(w180) -> ()
              n6431 = local write "单选_第45路"(w180) -> ()
              n6432 = local write "单选_第46路"(w180) -> ()
              n6433 = local write "单选_第47路"(w180) -> ()
              n6434 = local write "单选_第48路"(w180) -> ()
              n6435 = local write "单选_第49路"(w180) -> ()
              n6436 = local write "单选_第50路"(w180) -> ()
              n6437 = local write "单选_第51路"(w180) -> ()
              n6438 = local write "单选_第52路"(w180) -> ()
              n6439 = local write "单选_第53路"(w180) -> ()
              n6440 = local write "单选_第54路"(w180) -> ()
              n6441 = local write "单选_第55路"(w180) -> ()
              n6442 = local write "单选_第56路"(w180) -> ()
              n6443 = local write "单选_第57路"(w180) -> ()
              n6444 = local write "单选_第58路"(w180) -> ()
              n6445 = local write "单选_第59路"(w180) -> ()
              n6446 = local write "单选_第60路"(w180) -> ()
              n6447 = local write "单选_第71路"(w180) -> ()
              n6448 = local write "单选_第79路"(w180) -> ()
              n6449 = local write "单选_第65路"(w180) -> ()
              n6450 = local write "单选_第66路"(w180) -> ()
              n6451 = local write "单选_第67路"(w180) -> ()
              n6452 = local write "单选_第68路"(w180) -> ()
              n6453 = local write "单选_第69路"(w180) -> ()
              n6454 = local write "单选_第70路"(w180) -> ()
              n6455 = local write "单选_第72路"(w180) -> ()
              n6456 = local write "单选_第73路"(w180) -> ()
              n6457 = local write "单选_第74路"(w180) -> ()
              n6458 = local write "单选_第75路"(w180) -> ()
              n6459 = local write "单选_第76路"(w180) -> ()
              n6460 = local write "单选_第77路"(w180) -> ()
              n6461 = local write "单选_第78路"(w180) -> ()
              n6462 = local write "单选_第80路"(w180) -> ()
            }
          }
        }
      }
    }
    frame #1 {
      w185 = "DOCheckStart" ("名称（未命名）")
      w188 = "DOStart" ("名称（未命名）")
      n6463 = while {
        stop <- w536 stop-if-true
        n6464 = event shown="[15] \"btn_全选\": 值改变" {
          selector: _ -> [_ _ _ _ _ _ _ _ _ _ _ _ _ _ _ _ _ _ _]
          dyn-events: _ -> [_ _ _ _ _ _ _ _ _ _ _ _ _ _ _ _ _ _ _]
          timeout: _ -> [_ _ _ _ _ _ _ _ _ _ _ _ _ _ _ _ _ _ _]
          tunnel: [_ w537 w538 _ _ _ _ _ _ _ _ _ _ _ _ _ _ _ _] -> w536
          event Timeout {
            n6465 = event-data() -> ()  [unwired: 1 in, 2 out]
          }
          event Panel Close {
            w537 = TRUE ("关闭？")
            n6466 = event-data() -> ()  [unwired: 1 in, 3 out]
            n6467 = local write "关闭？"(w537) -> ()
          }
          event "btn_关闭": Value Change {
            w538 = TRUE
            n6468 = event-data() -> ()  [unwired: 1 in, 5 out]
            n6469 = local write "关闭？"(w538) -> ()
          }
          event "btn_全选_1": Value Change {
            n6470 = event-data() -> ("NewVal"=w540:bool)  [unwired: 1 in, 4 out]
            n6471 = case shown="假" w540 {
              tunnel: [FALSE ("单选_第41路") TRUE ("单选_第41路")] -> w539
              frame False {
              }
              frame True {
              }
            }
            n6472 = local write "单选_第1路"(w539) -> ()
            n6473 = local write "单选_第2路"(w539) -> ()
            n6474 = local write "单选_第3路"(w539) -> ()
            n6475 = local write "单选_第4路"(w539) -> ()
            n6476 = local write "单选_第5路"(w539) -> ()
            n6477 = local write "单选_第6路"(w539) -> ()
            n6478 = local write "单选_第7路"(w539) -> ()
            n6479 = local write "单选_第8路"(w539) -> ()
            n6480 = local write "单选_第9路"(w539) -> ()
            n6481 = local write "单选_第10路"(w539) -> ()
            n6482 = local write "单选_第11路"(w539) -> ()
            n6483 = local write "单选_第12路"(w539) -> ()
            n6484 = local write "单选_第13路"(w539) -> ()
            n6485 = local write "单选_第14路"(w539) -> ()
            n6486 = local write "单选_第15路"(w539) -> ()
            n6487 = local write "单选_第16路"(w539) -> ()
          }
          event "btn_全选_2": Value Change {
            n6488 = event-data() -> ("NewVal"=w544:bool)  [unwired: 1 in, 4 out]
            n6489 = case shown="假" w544 {
              tunnel: [FALSE ("单选_第41路") TRUE ("单选_第41路")] -> w543
              frame False {
              }
              frame True {
              }
            }
            n6490 = local write "单选_第17路"(w543) -> ()
            n6491 = local write "单选_第18路"(w543) -> ()
            n6492 = local write "单选_第19路"(w543) -> ()
            n6493 = local write "单选_第20路"(w543) -> ()
            n6494 = local write "单选_第21路"(w543) -> ()
            n6495 = local write "单选_第22路"(w543) -> ()
            n6496 = local write "单选_第23路"(w543) -> ()
            n6497 = local write "单选_第24路"(w543) -> ()
            n6498 = local write "单选_第25路"(w543) -> ()
            n6499 = local write "单选_第26路"(w543) -> ()
            n6500 = local write "单选_第27路"(w543) -> ()
            n6501 = local write "单选_第28路"(w543) -> ()
            n6502 = local write "单选_第29路"(w543) -> ()
            n6503 = local write "单选_第30路"(w543) -> ()
            n6504 = local write "单选_第31路"(w543) -> ()
            n6505 = local write "单选_第32路"(w543) -> ()
          }
          event "btn_全选_3": Value Change {
            n6506 = event-data() -> ("NewVal"=w548:bool)  [unwired: 1 in, 4 out]
            n6507 = case shown="假" w548 {
              tunnel: [FALSE ("单选_第41路") TRUE ("单选_第41路")] -> w547
              frame False {
              }
              frame True {
              }
            }
            n6508 = local write "单选_第33路"(w547) -> ()
            n6509 = local write "单选_第34路"(w547) -> ()
            n6510 = local write "单选_第35路"(w547) -> ()
            n6511 = local write "单选_第36路"(w547) -> ()
            n6512 = local write "单选_第37路"(w547) -> ()
            n6513 = local write "单选_第38路"(w547) -> ()
            n6514 = local write "单选_第39路"(w547) -> ()
            n6515 = local write "单选_第40路"(w547) -> ()
            n6516 = local write "单选_第41路"(w547) -> ()
            n6517 = local write "单选_第42路"(w547) -> ()
            n6518 = local write "单选_第43路"(w547) -> ()
            n6519 = local write "单选_第44路"(w547) -> ()
            n6520 = local write "单选_第45路"(w547) -> ()
            n6521 = local write "单选_第46路"(w547) -> ()
            n6522 = local write "单选_第47路"(w547) -> ()
            n6523 = local write "单选_第48路"(w547) -> ()
          }
          event "btn_全选_4": Value Change {
            n6524 = event-data() -> ("NewVal"=w552:bool)  [unwired: 1 in, 4 out]
            n6525 = case shown="假" w552 {
